vi "SHA-1 Hash.vi"(2 "Message (\"\")":string) -> (0 "SHA-1 Hash":string)   [LabVIEW 2011]
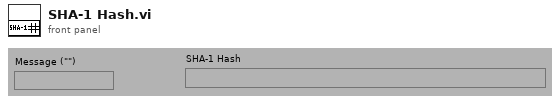
[diagram p1: front panel]
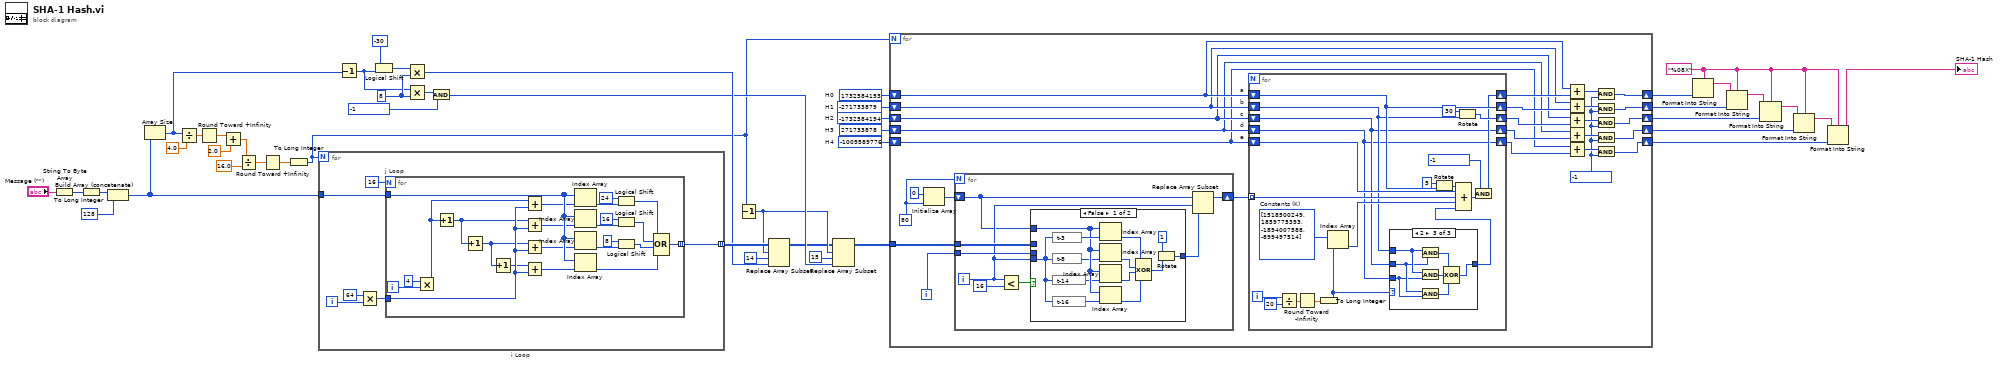
[diagram p0: block diagram]
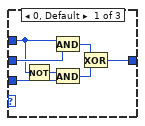
[diagram p2: hidden frame]
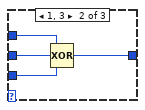
[diagram p3: hidden frame]
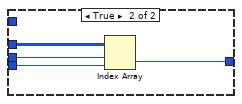
[diagram p4: hidden frame]
diagram:
  w13 = "%08X"
  w20 = -1009589776  # H4
  w21 = 271733878  # H3
  w22 = -1732584194  # H2
  w23 = -271733879  # H1
  w24 = 1732584193  # H0
  w33 = 8 ("x-1")
  n1 = String To Byte Array(string="Message (\"\")") -> (unsigned byte array=w36:u8[])
  n2 = To Long Integer(number=w36) -> (32bit integer=w6:i32[])
  n3 = Build Array (concatenate)(w6, 128) -> (w7:i32[])
  n4 = Array Size(array=w7) -> (size(s)=w8:i32)
  n5 = Divide(x=w8, y=4.0) -> (x/y=w43:dbl)
  n6 = Round Toward +Infinity(x=w43) -> (ceil(x): smallest int >= x=w39:dbl)
  n7 = Add(x=w39, y=2.0) -> (x+y=w41:dbl)
  n8 = Divide(x=w41, y=16.0) -> (x/y=w38:dbl)
  n9 = Round Toward +Infinity(x=w38) -> (ceil(x): smallest int >= x=w37:dbl)
  n10 = To Long Integer(number=w37) -> (32bit integer=w19:i32)
  n11 = for "i Loop" {
    N: w19 -> [_]
    tunnel: w7 -> [w51]
    tunnel: [w46] -> w30 mode=indexing
    i -> [w49]
    n12 = Multiply(x=64, y=w49) -> (x*y=w47:i32)
    n13 = for "j Loop" {
      N: 16 -> [_]
      tunnel: w51 -> [w74]
      tunnel: w47 -> [w72]
      tunnel: [w71] -> w46 mode=indexing
      i -> [w58]
      n14 = Multiply(x=4, y=w58) -> (x*y=w57:i32)
      n15 = Increment(x=w57) -> (x+1=w56:i32)
      n16 = Increment(x=w56) -> (x+1=w55:i32)
      n17 = Increment(x=w55) -> (x+1=w54:i32)
      n18 = Add(x=w57, y=w72) -> (x+y=w69:i32)
      n19 = Add(x=w56, y=w72) -> (x+y=w68:i32)
      n20 = Add(x=w55, y=w72) -> (x+y=w67:i32)
      n21 = Add(x=w54, y=w72) -> (x+y=w70:i32)
      n22 = Index Array(array=w74, index=w69) -> (element=w63:i32)
      n23 = Index Array(array=w74, index=w68) -> (element=w62:i32)
      n24 = Index Array(array=w74, index=w67) -> (element=w61:i32)
      n25 = Index Array(array=w74, index=w70) -> (element=w52:i32)
      n26 = Logical Shift(y=24 ("x"), x=w63) -> (x << y=w60:i32)
      n27 = Logical Shift(y=16 ("x"), x=w62) -> (x << y=w59:i32)
      n28 = Logical Shift(y=8 ("x"), x=w61) -> (x << y=w53:i32)
      n29 = Compound Arithmetic op=OR(w60, w59, w53, w52) -> (w71:i32)
    }
  }
  n30 = Decrement(x=w8) -> (x-1=w16:i32)
  n31 = Logical Shift(y=-30 ("x"), x=w16) -> (x << y=w34:i32)
  n32 = Multiply(x=w34, y=w33) -> (x*y=w27:i32)
  n33 = Multiply(x=w16, y=w33) -> (x*y=w32:i32)
  n34 = And(x=w32, y=-1) -> (x .and. y?=w26:i32)
  n35 = Decrement(x=w19) -> (x-1=w25:i32)
  n36 = Replace Array Subset(array=w30, new element=w27, index (row)=w25, index (col)=14 ("disabled index (col)")) -> (w18:i32[][])
  n37 = Replace Array Subset(array=w18, new element=w26, index (row)=w25, index (col)=15 ("disabled index (col)")) -> (w17:i32[][])
  n38 = for {
    N: w19 -> [_]
    shift-right: [w94] -> w14
    shift-left: w24 -> [w79]
    shift-right: [w90] -> w12
    shift-left: w23 -> [w78]
    shift-right: [w84] -> w11
    shift-left: w22 -> [w77]
    shift-right: [w83] -> w10
    shift-left: w21 -> [w76]
    shift-right: [w80] -> w9
    shift-left: w20 -> [w75]
    tunnel: w17 -> [w101]
    i -> [w100]
    w82 = -1
    w97 = 80
    # "e"
    # "d"
    # "c"
    # "b"
    # "a"
    n39 = Initialize Array(0, w97) -> (w98:i32[])
    n40 = for {
      N: w97 -> [_]
      tunnel: w101 -> [w147]
      tunnel: w100 -> [w146]
      shift-right: [w143] -> w96
      shift-left: w98 -> [w141]
      i -> [w145]
      n41 = Less?(x=w145, y=16) -> (x < y?=w142:bool)
      n42 = case shown="False" w142 {
        tunnel: w147 -> [_ w165]
        tunnel: w146 -> [_ w164]
        tunnel: w145 -> [w159 w163]
        tunnel: [w151 w162] -> w144
        tunnel: w141 -> [w158 _]
        frame False {
          n43 = expression code="t-3"(w159) -> (w160:i32)
          n44 = expression code="t-8"(w159) -> (w157:i32)
          n45 = expression code="t-14"(w159) -> (w156:i32)
          n46 = expression code="t-16"(w159) -> (w155:i32)
          n47 = Index Array(array=w158, index=w160) -> (element=w161:i32)
          n48 = Index Array(array=w158, index=w157) -> (element=w154:i32)
          n49 = Index Array(array=w158, index=w156) -> (element=w153:i32)
          n50 = Index Array(array=w158, index=w155) -> (element=w152:i32)
          n51 = Compound Arithmetic op=XOR(w161, w154, w153, w152) -> (w150:i32)
          n52 = Rotate(1:w150, 2:1 ("y")) -> (0:w151:i32)
        }
        frame True {
          n53 = Index Array(array=w165, index (row)=w164, index (col)=w163) -> (element=w162:i32)
        }
      }
      n54 = Replace Array Subset(array=w141, new element=w144, index=w145) -> (w143:i32[])
    }
    n55 = for {
      tunnel: w96 -> [w110] mode=indexing
      shift-right: [w107] -> w95
      shift-left: w79 -> [w119]
      shift-right: [w119] -> w91
      shift-left: w78 -> [w105]
      shift-right: [w121] -> w87
      shift-left: w77 -> [w104]
      shift-right: [w104] -> w86
      shift-left: w76 -> [w103]
      shift-right: [w103] -> w81
      shift-left: w75 -> [w117]
      i -> [w115]
      w116 = i32[] [1518500249, 1859775393, -1894007588, -899497514]  # Constants (K)
      n56 = Divide(x=w115, y=20) -> (x/y=w113:dbl)
      n57 = Round Toward -Infinity(1:w113) -> (0:w112:dbl)
      n58 = To Long Integer(number=w112) -> (32bit integer=w106:i32)
      n59 = Index Array(array=w116, index=w106) -> (element=w111:i32)
      n60 = case shown="2" w106 {
        tunnel: w105 -> [w126 w133 w140]
        tunnel: w104 -> [w129 w132 w139]
        tunnel: w103 -> [w128 w131 w138]
        tunnel: [w123 w130 w134] -> w102
        frame 0, Default {
          n61 = Not(x=w126) -> (.not. x?=w127:i32)
          n62 = And(x=w126, y=w129) -> (x .and. y?=w125:i32)
          n63 = And(x=w127, y=w128) -> (x .and. y?=w124:i32)
          n64 = Exclusive Or(1:w124, 2:w125) -> (0:w123:i32)
        }
        frame 1, 3 {
          n65 = Compound Arithmetic op=XOR(w133, w132, w131) -> (w130:i32)
        }
        frame 2 {
          n66 = And(x=w140, y=w139) -> (x .and. y?=w136:i32)
          n67 = And(x=w140, y=w138) -> (x .and. y?=w137:i32)
          n68 = And(x=w139, y=w138) -> (x .and. y?=w135:i32)
          n69 = Compound Arithmetic op=XOR(w136, w137, w135) -> (w134:i32)
        }
      }
      n70 = Rotate(1:w119, 2:5 ("y")) -> (0:w118:i32)
      n71 = Compound Arithmetic op=ADD(w118, w117, w110, w111, w102) -> (w109:i32)
      n72 = Rotate(1:w105, 2:30 ("y")) -> (0:w121:i32)
      n73 = And(x=-1, y=w109) -> (x .and. y?=w107:i32)
    }
    n74 = Add(x=w79, y=w95) -> (x+y=w93:i32)
    n75 = Add(x=w78, y=w91) -> (x+y=w92:i32)
    n76 = Add(x=w77, y=w87) -> (x+y=w88:i32)
    n77 = Add(x=w76, y=w86) -> (x+y=w89:i32)
    n78 = Add(x=w75, y=w81) -> (x+y=w85:i32)
    n79 = And(x=w93, y=w82) -> (x .and. y?=w94:i32)
    n80 = And(x=w92, y=w82) -> (x .and. y?=w90:i32)
    n81 = And(x=w88, y=w82) -> (x .and. y?=w84:i32)
    n82 = And(x=w89, y=w82) -> (x .and. y?=w83:i32)
    n83 = And(x=w85, y=w82) -> (x .and. y?=w80:i32)
  }
  n84 = Format Into String(format string=w13, w14) -> (resulting string=w5:string)  [unwired: 2 in, 1 out]
  n85 = Format Into String(format string=w13, initial string=w5, w12) -> (resulting string=w4:string)  [unwired: 1 in, 1 out]
  n86 = Format Into String(format string=w13, initial string=w4, w11) -> (resulting string=w3:string)  [unwired: 1 in, 1 out]
  n87 = Format Into String(format string=w13, initial string=w3, w10) -> (resulting string=w2:string)  [unwired: 1 in, 1 out]
  n88 = Format Into String(format string=w13, initial string=w2, w9) -> (resulting string=→"SHA-1 Hash":string)  [unwired: 1 in, 1 out]
